vi "AllFolderInfo.vi"(4 "error in (no error)":errorcluster, 5 "Root":path, 6 "Max digit of index":i32=4, 7 "Key words":string="Trace_") -> (0 "error out":errorcluster, 1 "Folder order correct? (Last mod : index)":bool, 2 "max value":i32, 3 "data folder info":T1 caption="Folder name                    Description                                                                              Folder index     Key words           Log in finding index")   [LabVIEW 2020, in "Initialization.lvlib" / "FileManagement.lvlib"]
uses:
  FileManagement.lvlib
  Folder information.ctl
  BasicVIs/BasicVIs.lvlib
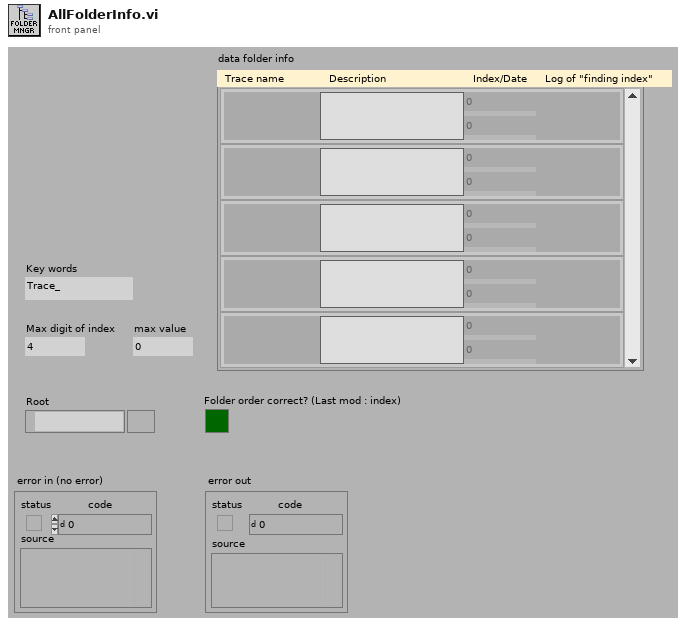
[diagram p1: front panel]
types:
  T1 = typedef "Initialization.lvlib/FileManagement.lvlib/Folder information.ctl" = cluster{"Folder index":i32, "Date modefied":i32, "Folder name":string, "Description":string, "Key words":string, "Log in Finding index":string}[]
  T2 = cluster{"Date modefied":i32, "Folder index":i32, "Folder name":string, "Description":string, "Key words":string, "Log in Finding index":string}[]
  T3 = cluster{"Folder index":i32, "Date modefied":i32, "Folder name":string, "Description":string, "Key words":string, "Log in Finding index":string}
  T4 = cluster{"Folder index":i32, "Date modefied":i32, "Folder name":string, "Description":string, "Key words":string, "Log in Finding index":string}[]
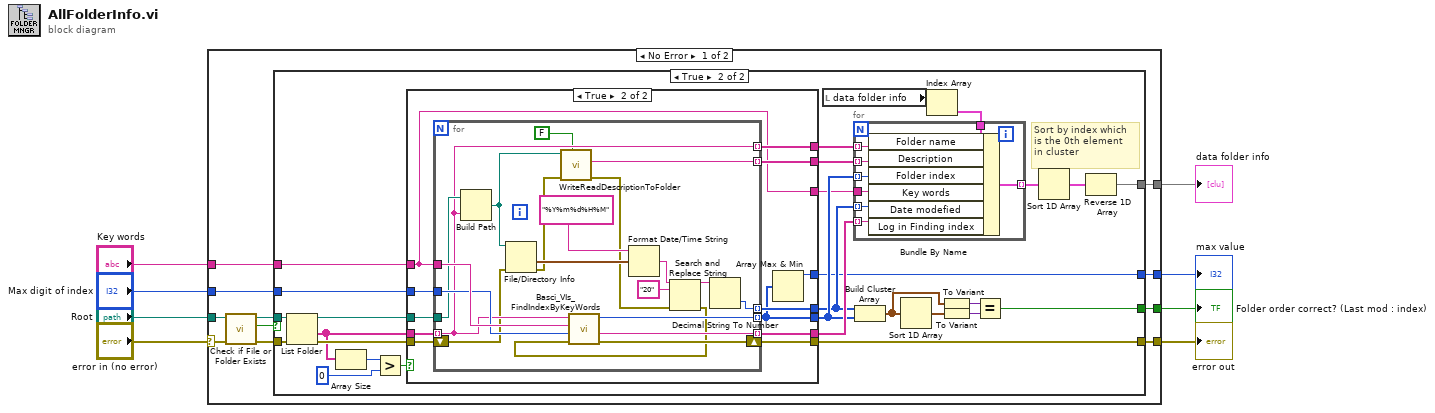
[diagram p0: block diagram]
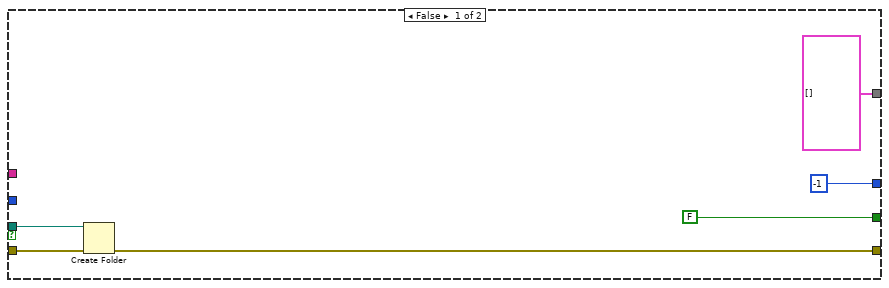
[diagram p2: hidden frame]
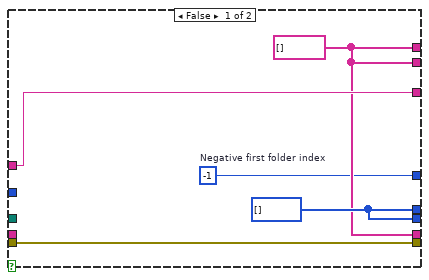
[diagram p3: hidden frame]
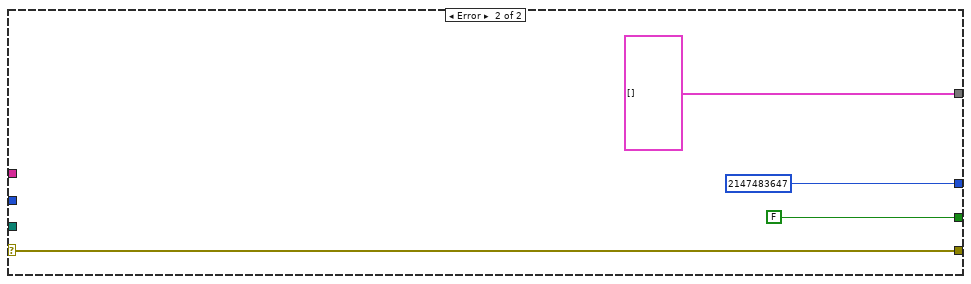
[diagram p4: hidden frame]
diagram:
  n1 = case shown="No Error" "error in (no error)" {
    selector: "error in (no error)" -> [w15 w102]
    tunnel: "Root" -> [w19 _]
    tunnel: "Key words" -> [w14 _]
    tunnel: "Max digit of index" -> [w10 _]
    tunnel: [w13 w102] -> w5
    tunnel: [w12 FALSE] -> w4
    tunnel: [w11 2147483647] -> w3
    tunnel: [w9 T2 []] -> w2
    frame No Error {
      n2 = call <vilib>:"Check if File or Folder Exists.vi"("error in (no error)"=w15, "path"=w19) -> ("error out"=w16:errorcluster, "file or folder exists?"=w18:bool, "dup path"=w17:path)  [unwired: 7 in]
      n3 = case shown="True" w18 {
        tunnel: w17 -> [w22 w53]
        tunnel: w16 -> [w23 w52]
        tunnel: w14 -> [_ w34]
        tunnel: w10 -> [_ w29]
        tunnel: [w21 w45] -> w13
        tunnel: [FALSE w44] -> w12
        tunnel: [-1 w28] -> w11
        tunnel: [T2 [] w31] -> w9
        frame False {
          n4 = Create Folder(path (use dialog)=w22, error in=w23) -> (error out=w21:errorcluster)  [unwired: 1 in, 2 out]
        }
        frame True {
          # "Sort by index which\nis the 0th element\nin cluster"
          n5 = List Folder(path=w53, error in=w52) -> (path out=w51:path, folder names=w38:string[], error out=w50:errorcluster)  [unwired: 2 in, 1 out]
          n6 = Array Size(array=w38) -> (size(s)=w37:i32)
          n7 = Greater?(x=w37, y=0) -> (0:w35:bool)
          n8 = case shown="True" w35 {
            tunnel: w38 -> [_ w70]
            tunnel: w29 -> [_ w69]
            tunnel: w51 -> [_ w68]
            tunnel: w50 -> [w58 w67]
            tunnel: [w58 w66] -> w45
            tunnel: [w55 w65] -> w43
            tunnel: [w56 w59] -> w42
            tunnel: [w55 w64] -> w41
            tunnel: [w55 w63] -> w40
            tunnel: [w56 w62] -> w39
            tunnel: w34 -> [w57 w61]
            tunnel: [w57 w61] -> w30
            tunnel: [w54 w60] -> w28
            frame False {
              w55 = string[] []
              w56 = i32[] []
              w54 = -1  # Negative first folder index
            }
            frame True {
              n9 = for {
                tunnel: w70 -> [w82] mode=indexing
                tunnel: w61 -> [w90]
                tunnel: w69 -> [w89]
                tunnel: w68 -> [w86]
                shift-right: [w81] -> w66
                shift-left: w67 -> [w80]
                tunnel: [w88] -> w59 mode=indexing
                tunnel: [w87] -> w65 mode=indexing
                tunnel: [w76] -> w62 mode=indexing
                tunnel: [w82] -> w63 mode=indexing
                tunnel: [w71] -> w64 mode=indexing
                n10 = Build Path(base path=w86, name or relative path=w82) -> (appended path=w75:path)
                n11 = File/Directory Info(path=w75, error in=w80) -> (last mod=w83:timestamp, error out=w73:errorcluster)  [unwired: 5 out]
                n12 = call "WriteReadDescriptionToFolder.vi"("F: Read/ T: Write (default)"=FALSE, "error in"=w73, "Folder path"=w75) -> ("error out"=w72:errorcluster, "Description for folder out"=w71:string)  [unwired: 2 in, 2 out]
                n13 = Format Date/Time String(time format string (%c)="%Y%m%d%H%M" ("时间格式字符串(%c)"), seconds (now)=w83) -> (date/time string=w78:string)  [unwired: 1 in]
                n14 = Search and Replace String(input string=w78, search string="20" ("substring (\"\")"), error in=w72) -> (result string=w77:string, error out=w79:errorcluster)  [unwired: 5 in, 2 out]
                n15 = call "Basci_VIs_FindIndexByKeyWords.vi"("error in (no error)"=w79, "Max length\nof index"=w89, "Key words"=w90, "String input"=w82) -> ("error out"=w81:errorcluster, "Log"=w87:string, "Folder index"=w88:i32)  [unwired: 1 out]
                n16 = Decimal String To Number(string=w77) -> (number=w76:i32)  [unwired: 2 in, 1 out]
              }
              n17 = Array Max & Min(array=w59) -> (max value=w60:i32)  [unwired: 3 out]
            }
          }
          n18 = local read "data folder info"() -> (w27:T1)
          n19 = Build Cluster Array(w39, w42) -> (w48:cluster{i32, "Folder index":i32}[])
          n20 = Sort 1D Array(array=w48) -> (sorted array=w49:cluster{i32, "Folder index":i32}[])
          n21 = Index Array(array=w27) -> (element=w26:T3)  [unwired: 1 in]
          n22 = for {
            tunnel: w43 -> [w91] mode=indexing
            tunnel: w42 -> [w94] mode=indexing
            tunnel: w41 -> [w96] mode=indexing
            tunnel: w40 -> [w97] mode=indexing
            tunnel: w39 -> [w92] mode=indexing
            tunnel: w26 -> [w98]
            tunnel: [w95] -> w33 mode=indexing
            tunnel: w30 -> [w93]
            n23 = Bundle By Name(cluster=w98, "Folder name"=w97, "Description"=w96, "Folder index"=w94, "Key words"=w93, "Date modefied"=w92, "Log in Finding index"=w91) -> (w95:T3)
          }
          n24 = To Variant(anything=w48) -> (Variant=w46:variant)
          n25 = To Variant(anything=w49) -> (Variant=w47:variant)
          n26 = Equal?(x=w46, y=w47) -> (x = y?=w44:bool)
          n27 = Sort 1D Array(array=w33) -> (sorted array=w32:T4)
          n28 = Reverse 1D Array(array=w32) -> (reversed array=w31:T4)
        }
      }
    }
    frame Error {
    }
  }
  "error out" <- w5
  "Folder order correct? (Last mod : index)" <- w4
  "max value" <- w3
  "data folder info" <- w2
